vi "isComplete.vi"(8 "error in (no error)":errorcluster, 11 "Mission in":refnum<class "Mission.lvclass">) -> (0 "error out":errorcluster, 2 "Mission Complete?":bool, 3 "Mission out":refnum<class "Mission.lvclass">)   [LabVIEW 2011, in "Mission.lvclass"]
uses:
  Mission.lvclass
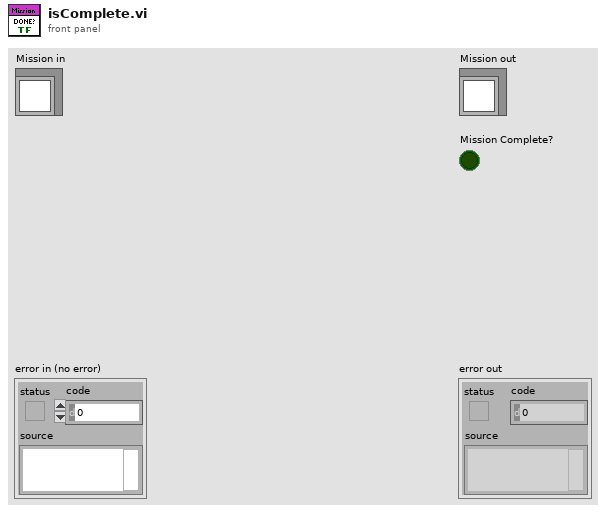
[diagram p1: front panel]
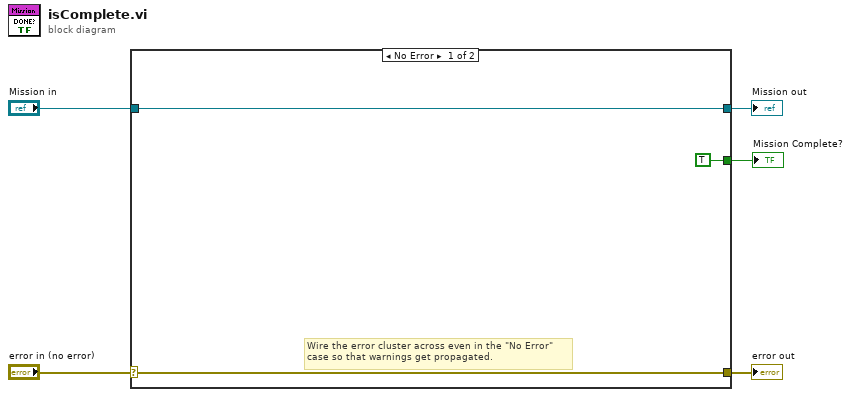
[diagram p0: block diagram]
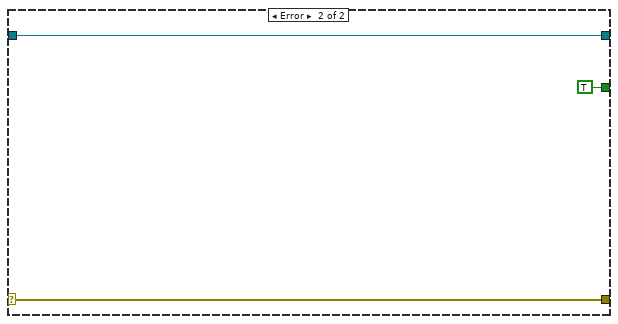
[diagram p2: hidden frame]
diagram:
  n1 = case shown="No Error" "error in (no error)" {
    selector: "error in (no error)" -> [w7 w11]
    tunnel: [w7 w11] -> w4
    tunnel: [w8 w10] -> w2
    tunnel: "Mission in" -> [w8 w10]
    tunnel: [TRUE ("Mission Complete?") TRUE ("Mission Complete?")] -> w1
    frame No Error {
      # "Wire the error cluster across even in the \"No Error\"\ncase so that warnings get propagated."
    }
    frame Error {
    }
  }
  "error out" <- w4
  "Mission out" <- w2
  "Mission Complete?" <- w1
